vi "Broken.vi"(11 "Dummy in":refnum<class "Example Test Case.lvclass">) -> (0 "error out":errorcluster, 3 "Dummy out":refnum<class "Example Test Case.lvclass">)   [LabVIEW 2020, in "Example Test Case.lvclass"]
doc: "Broken test method"
uses:
  Example Test Case.lvclass
  Example Test Case.lvclass/Example Test Case.ctl
  API/LUnit Test Case/LUnit Test Case.lvclass
  C:/git/astemes-lunit/source/API/LUnit Test Case/LUnit Test Case.lvclass
  C:/git/astemes-lunit/source/Core/Runnable/Runnable.lvclass
  C:/git/astemes-lunit/source/Examples/Basic Example/Dummy/Example Test Case.lvclass
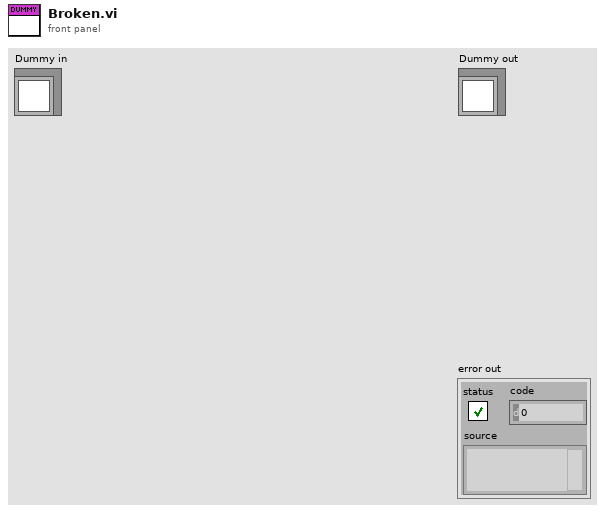
[diagram p1: front panel]
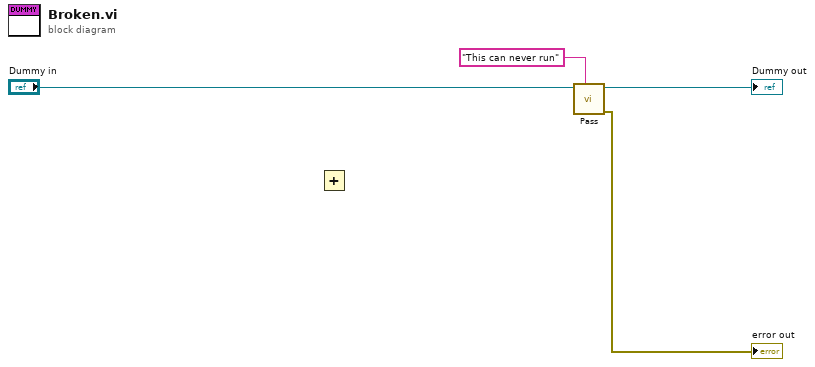
[diagram p0: block diagram]
diagram:
  n1 = Add() -> ()  [unwired: 2 in, 1 out]
  n2 = call "Pass.vi"("Description"="This can never run", "LUnit Test Case In"="Dummy in") -> ("error out"=→"error out":errorcluster, "LUnit Test Case Out"=→"Dummy out":refnum<class "Example Test Case.lvclass">)  [unwired: 8 in]
